vi "Enable Watchdog.vi"(8 "error in (no error)":errorcluster, 9 "Watchdog Delay (1)":u32=1 min=1 max=3600 step=1, 10 "Watchdog State (Off)":bool, 11 "VISA resource name":refnum<visa-resource-name>) -> (0 "error out":errorcluster, 3 "VISA resource name out":refnum<visa-resource-name>)   [LabVIEW 2017, in "HH PLI Series.lvlib"]
doc: "Enables or disables the watchdog. In case of a missing communication between the load and the computer the load disables the input."
uses:
  HH PLI Series.lvlib
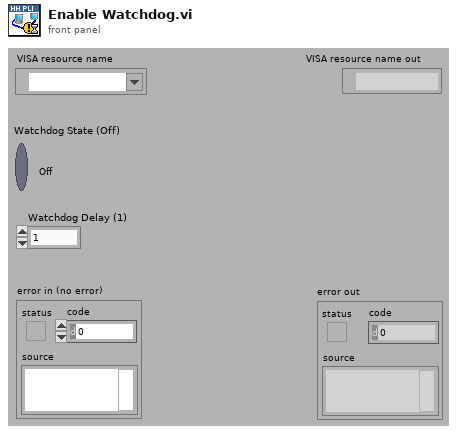
[diagram p1: front panel]
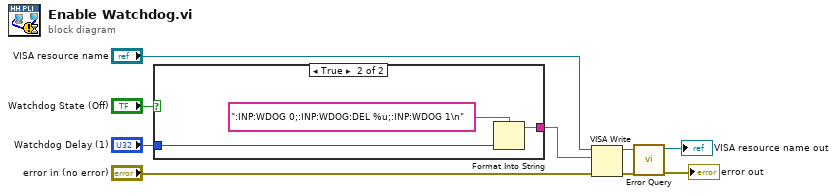
[diagram p0: block diagram]
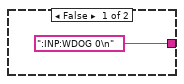
[diagram p2: hidden frame]
diagram:
  n1 = case shown="True" "Watchdog State (Off)" {
    tunnel: [":INP:WDOG 0\n" w12] -> w9
    tunnel: "Watchdog Delay (1)" -> [_ w11]
    frame False {
    }
    frame True {
      n2 = Format Into String(format string=":INP:WDOG 0;:INP:WDOG:DEL %u;:INP:WDOG 1\n", w11) -> (resulting string=w12:string)  [unwired: 2 in, 1 out]
    }
  }
  n3 = VISA Write(VISA resource name="VISA resource name", write buffer=w9, error in (no error)="error in (no error)") -> (VISA resource name out=w3:refnum<visa-resource-name>, error out=w4:errorcluster)  [unwired: 1 out]
  n4 = call "Error Query.vi"("error in (no error)"=w4, "VISA resource name"=w3) -> ("error out"=→"error out":errorcluster, "VISA resource name out"=→"VISA resource name out":refnum<visa-resource-name>)  [unwired: 6 in, 2 out]
